vi "Adjust Velocities w Interp.vi"(8 "Position In":cluster{"x":dbl, "y":dbl, "th":dbl}, 9 "Robot Velocities In":T1, 10 "ChoreoSwerveSample":T2, 11 "Choreo Traj?":bool) -> (2 "Position Out":cluster{"x":dbl, "y":dbl, "th":dbl}, 3 "Robot Velocities Out":T1)   [LabVIEW 2025]
uses:
  <vilib>/Rock Robotics/WPI/ThirdParty/ChoreoLib/TypeDef/ChoreoSwerveSample.ctl
  swerve-template/Type Definitions/Data/Robot Velocities.ctl
  <vilib>/Rock Robotics/WPI/ThirdParty/ChoreoLib/ChoreoLib.lvlib
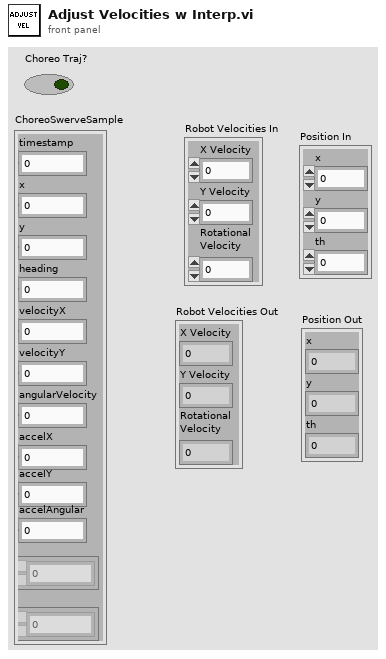
[diagram p1: front panel]
types:
  T1 = typedef "Robot Velocities.ctl" = cluster{"X Velocity":dbl, "Y Velocity":dbl, "Rotational \nVelocity":dbl}
  T2 = typedef "ChoreoLib.lvlib/ChoreoSwerveSample.ctl" = cluster{"timestamp":dbl, "x":dbl, "y":dbl, "heading":dbl, "velocityX":dbl, "velocityY":dbl, "angularVelocity":dbl, "accelX":dbl, "accelY":dbl, "accelAngular":dbl, "forceX":dbl[], "forceY":dbl[]}
  T3 = cluster{"velocityX":dbl, "velocityY":dbl, "angularVelocity":dbl}
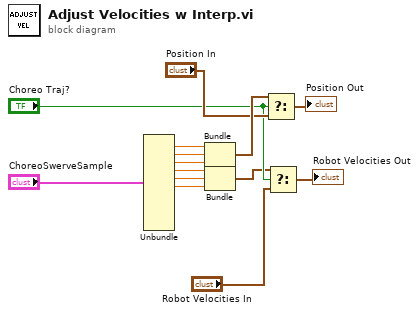
[diagram p0: block diagram]
diagram:
  n1 = Unbundle("ChoreoSwerveSample") -> ("x"=w13:dbl, "y"=w12:dbl, "heading"=w11:dbl, "velocityX"=w7:dbl, "velocityY"=w6:dbl, "angularVelocity"=w5:dbl)  [unwired: 6 out]
  n2 = Bundle("x"=w13, "y"=w12, "heading"=w11) -> (w10:cluster{"x":dbl, "y":dbl, "heading":dbl})  [unwired: 1 in]
  n3 = Bundle("velocityX"=w7, "velocityY"=w6, "angularVelocity"=w5) -> (w3:T3)  [unwired: 1 in]
  n4 = Select(t=w10, s="Choreo Traj?", f="Position In") -> (s? t:f=→"Position Out":cluster{"x":dbl, "y":dbl, "th":dbl})
  n5 = Select(t=w3, s="Choreo Traj?", f="Robot Velocities In") -> (s? t:f=→"Robot Velocities Out":T1)
